vi "TRACK set.vi"(7 "Track Mode":u16(ring) items=["Independent", "Series", "Parallel"], 8 "error in (no error)":errorcluster, 11 "VISA resource name":refnum<visa-resource-name>) -> (0 "error out":errorcluster, 3 "VISA resource name out":refnum<visa-resource-name>)   [LabVIEW 2020, in "GPP.lvlib"]
uses:
  GPP.lvlib
  Function/VISA_COMMON.ctl
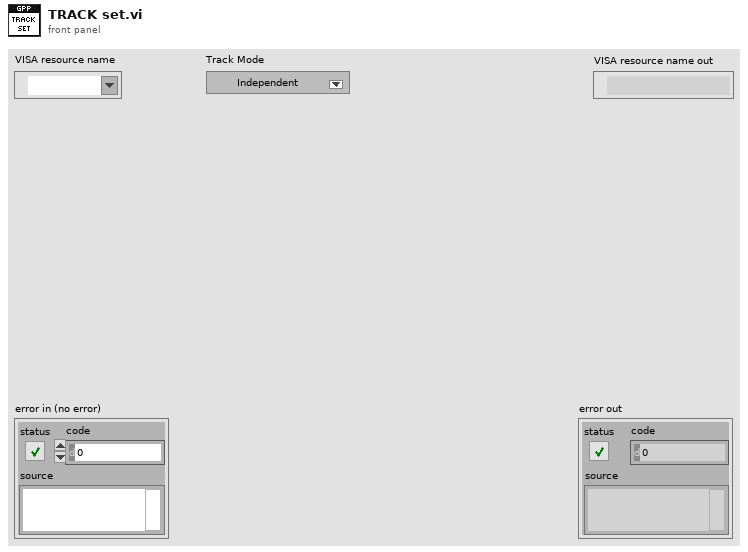
[diagram p1: front panel]
types:
  T1 = typedef "GPP.lvlib/VISA_COMMON.ctl" = enum16{"Initial", "Write CMD", "Read Result", "Read History", "Close"}
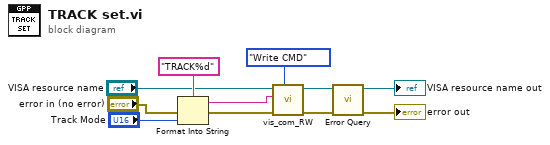
[diagram p0: block diagram]
diagram:
  n1 = Format Into String(format string="TRACK%d", error in="error in (no error)", "Track Mode") -> (resulting string=w5:string, error out=w6:errorcluster)  [unwired: 1 in]
  n2 = call "vis_com_RW.vi"("Funciton"=VISA_COMMON."Write CMD", "error in (no error)"=w6, "CMD String"=w5, "VISA resource in"="VISA resource name") -> ("error out"=w8:errorcluster, "VISA resource out"=w7:refnum<visa-resource-name>)  [unwired: 5 in, 1 out]
  n3 = call "Error Query.vi"("error in (no error)"=w8, "VISA resource name"=w7) -> ("error out"=→"error out":errorcluster, "VISA resource name out"=→"VISA resource name out":refnum<visa-resource-name>)  [unwired: 6 in, 2 out]
